vi "Set Reference.vi"(8 "ErrorIn":errorcluster, 10 "Reference":refnum<class "IRef.lvclass">, 11 "TopModuleIn":refnum<class "TopModule.lvclass">) -> (0 "ErrorOut":errorcluster, 3 "TopModuleOut":refnum<class "TopModule.lvclass">)   [LabVIEW 2020, in "TopModule.lvclass"]
uses:
  TopModule.lvclass
  IReference/IRef.lvclass
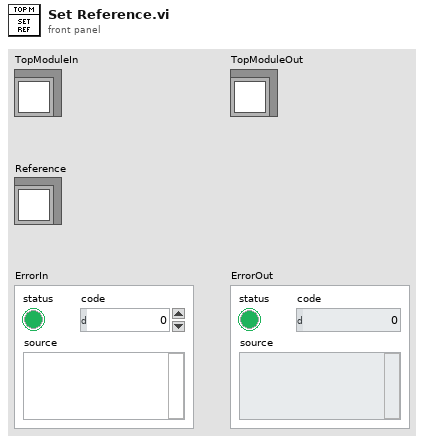
[diagram p1: front panel]
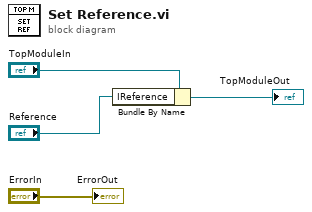
[diagram p0: block diagram]
diagram:
  n1 = Bundle By Name(cluster="TopModuleIn", "IReference"="Reference") -> (→"TopModuleOut":refnum<class "TopModule.lvclass">)
  "ErrorOut" <- "ErrorIn"
